vi "sub_rplidar_main.vi"(8 "error in":errorcluster) -> (0 "error out":errorcluster)   [LabVIEW 2019]
uses:
  Ctrl/rplidar_cmd.ctl
panel:
  out "buff chart":u32(graph)
  out "dt":u32
  out "i-2":i32
  out "i-1":i32
  out "XY 그래프":cluster{"X":dbl, "Y":dbl}[](graph)
  out "read buffer":string
  out "n in queue":i32
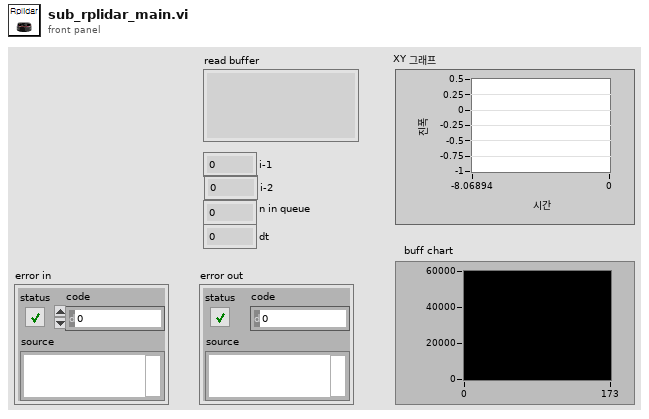
[diagram p1: front panel]
types:
  T1 = typedef "rplidar_cmd.ctl" = enum16{"init", "health", "spin", "scan", "read", "stop", "close"}
  T2 = cluster{"port":refnum<visa-resource-name>, "dt":u32, "update n":u8, "speed":u16, "rate ":u32}
  T3 = typedef "status.ctl" = u16
  T4 = cluster{"AGV":T3, "AGV Estop":T3, "Obstacle":T3, "Heading":T3, "Waypt":T3, "GNSS":T3, "VLP16":T3, "Cam":T3, "RPLidar":T3, "Joystick":T3}
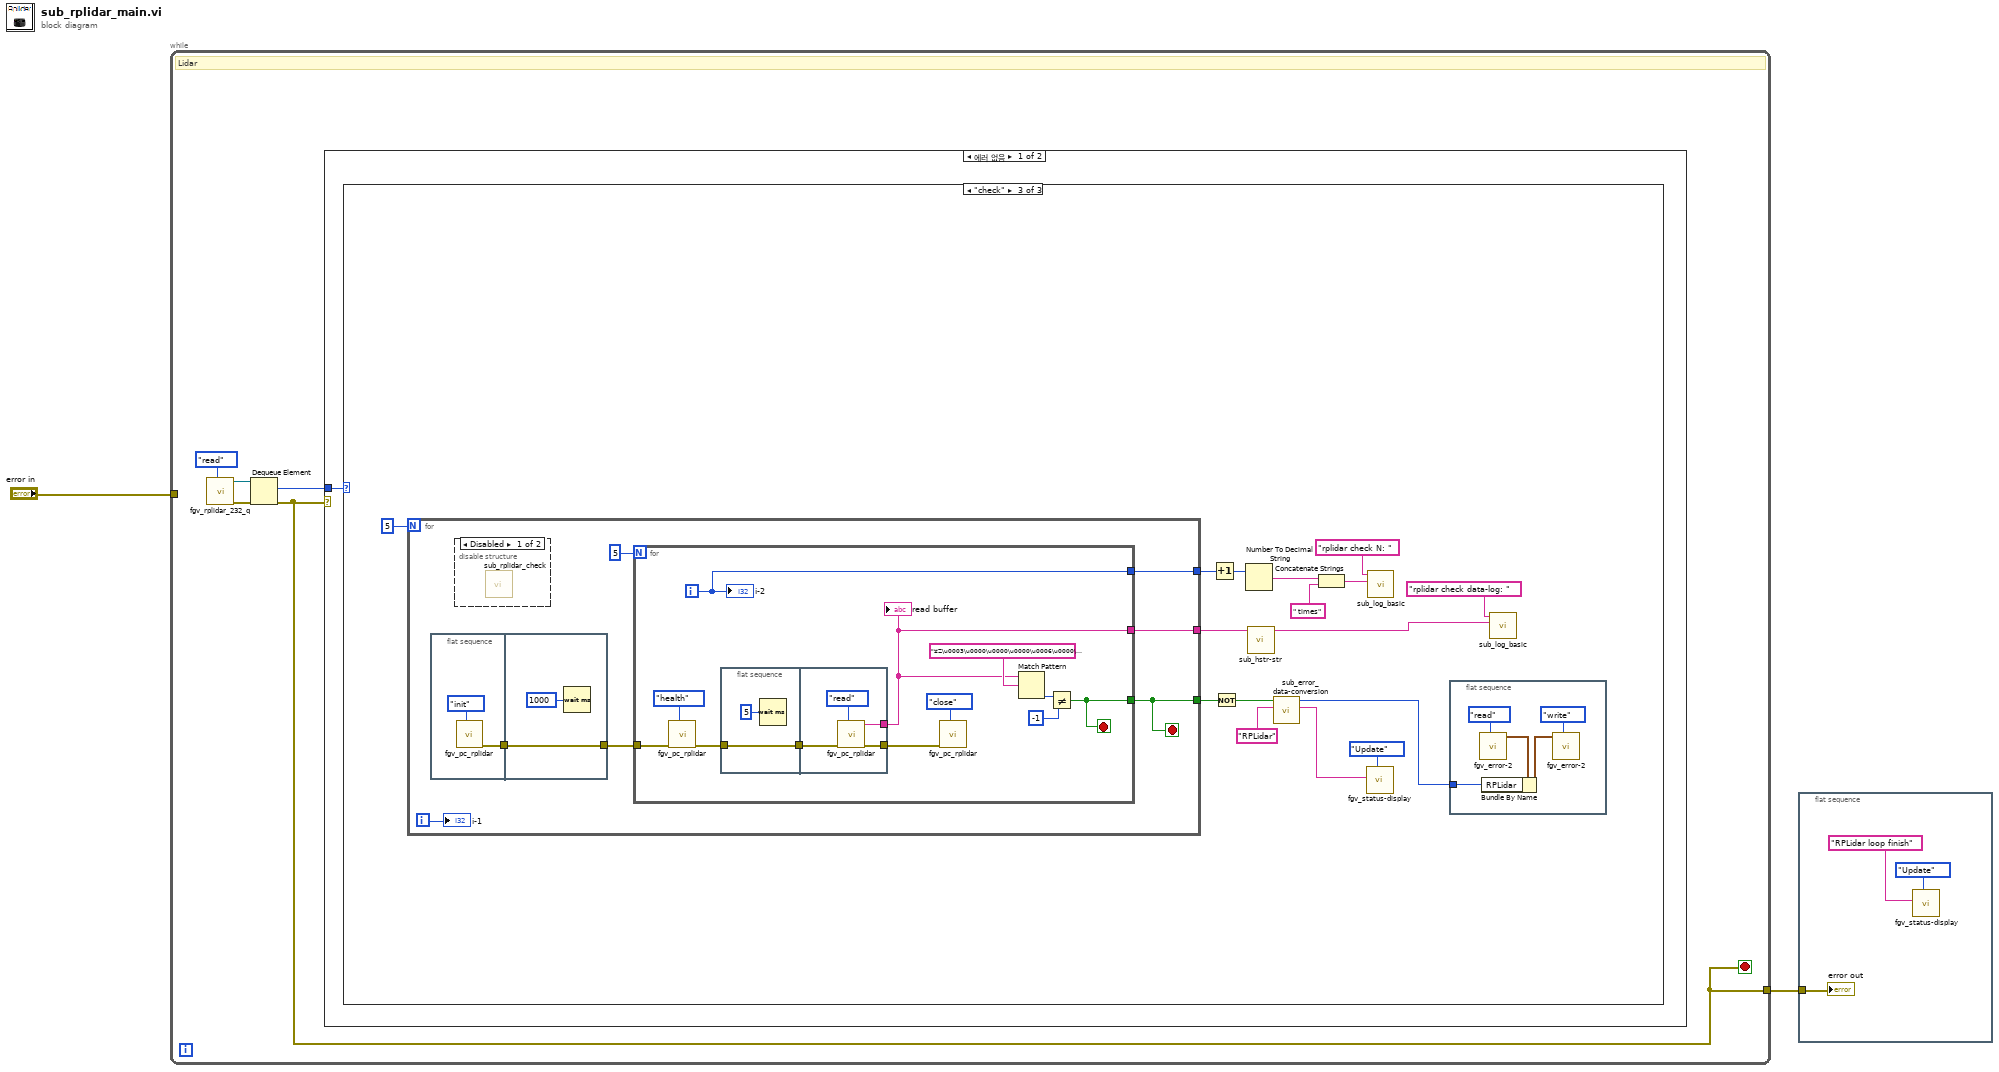
[diagram p0: block diagram]
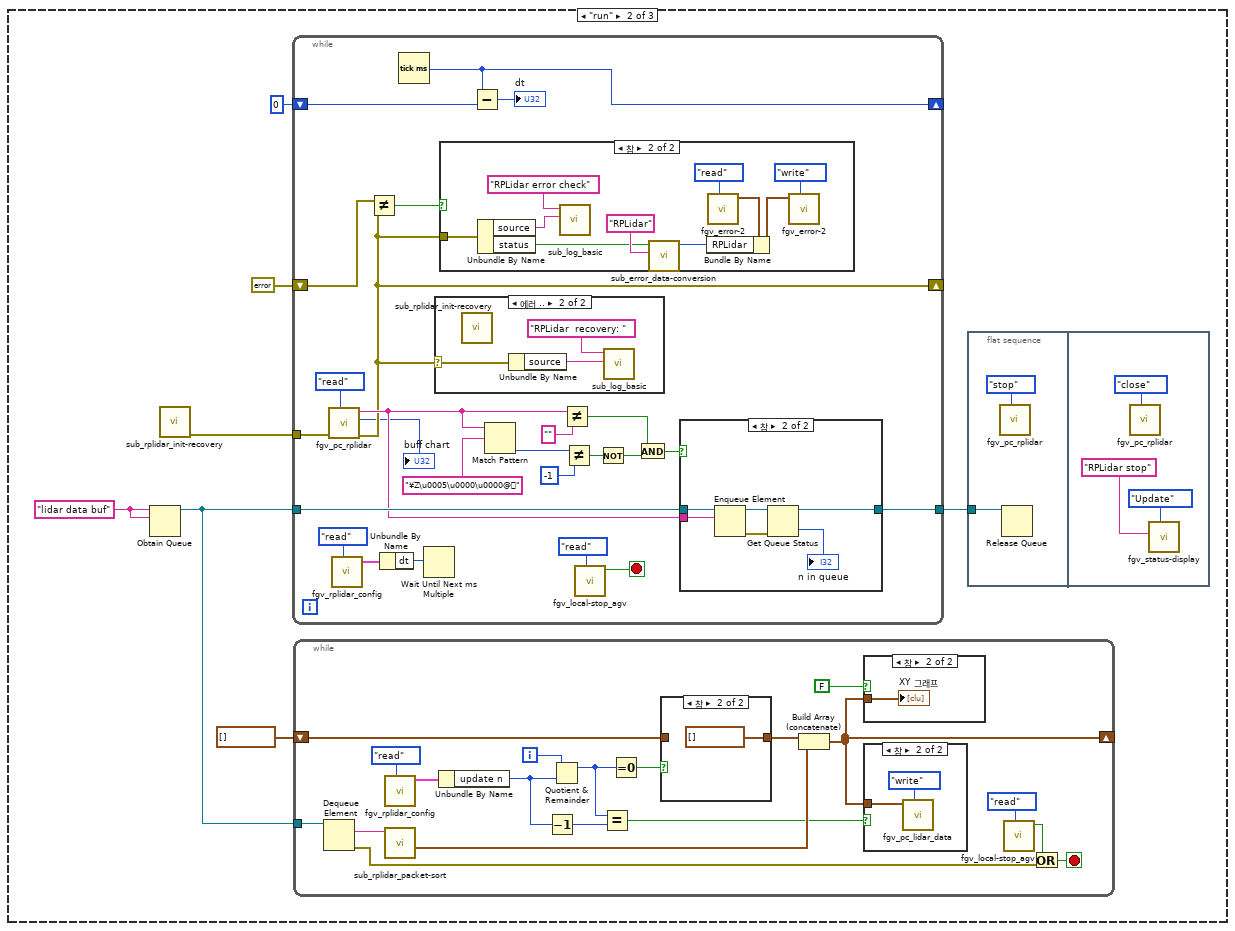
[diagram p3: hidden frame]
diagram:
  n1 = while {
    tunnel: "error in" -> [_]
    tunnel: [w3] -> w1
    stop <- w3 stop-if-true
    # "Lidar"
    n2 = call "fgv_rplidar_232_q.vi"("cmd"=enum16{"create", "write", "read", "close"}."read") -> ("error out"=w7:errorcluster, "queue out"=w4:refnum<queue>)  [unwired: 9 in]
    n3 = Dequeue Element(queue=w4, error in (no error)=w7) -> (element=w6:enum16{"run", "check", "stop"}, error out=w3:errorcluster)  [unwired: 1 in, 2 out]
    n4 = case shown="에러 없음" w3 {
      tunnel: w6 -> [w8 _]
      frame No Error {
        n5 = case shown="\"check\"" w8 {
          frame "stop", Default {
          }
          frame "run" {
            w15 = "lidar data buf" ("name (unnamed)")
            n6 = Obtain Queue(name (unnamed)=w15, element data type=w15) -> (queue out=w11:refnum<queue>)  [unwired: 3 in, 2 out]
            n7 = call "sub_rplidar_init-recovery.vi"() -> ("error out"=w14:errorcluster)  [unwired: 11 in]
            n8 = while {
              tunnel: w14 -> [w68]
              tunnel: w11 -> [w59]
              tunnel: [w58] -> w13
              shift-right: [w49] -> _
              shift-left: errorcluster {"status"=FALSE, "code"=0, "source"=""} ("error out") -> [w51]
              shift-right: [w47] -> _
              shift-left: u32 0 ("millisecond timer value") -> [w48]
              stop <- w55 stop-if-true
              n9 = call "fgv_pc_rplidar.vi"("cmd"=rplidar_cmd."read", "error in"=w68) -> ("error out"=w49:errorcluster, "serial buf"=→"buff chart":u32, "read buffer"=w57:string)  [unwired: 7 in]
              n10 = call "fgv_rplidar_config.vi"("cmd"=enum16{"read", "write"}."read") -> ("RPLidar cfg out"=w53:T2)  [unwired: 9 in, 1 out]
              n11 = Not Equal?(x=w51, y=w49) -> (x != y?=w50:bool)
              n12 = Unbundle By Name(w53) -> ("dt"=w52:u32)
              n13 = Tick Count (ms)() -> (millisecond timer value=w47:u32)
              n14 = Wait Until Next ms Multiple(millisecond multiple=w52) -> ()  [unwired: 1 out]
              n15 = case shown="에러 .." w49 {
                selector: w49 -> [_ w81]
                frame No Error {
                }
                frame Error {
                  n16 = call "sub_rplidar_init-recovery.vi"() -> ()  [unwired: 11 in, 1 out]
                  n17 = Unbundle By Name(w81) -> ("source"=w80:string)
                  n18 = call "sub_log_basic.vi"("desc"=w80, "Title"="RPLidar  recovery: ") -> ()  [unwired: 9 in, 1 out]
                }
              }
              n19 = case shown="참" w50 {
                tunnel: w49 -> [_ w78]
                frame False {
                }
                frame True {
                  n20 = Unbundle By Name(w78) -> ("source"=w70:string, "status"=w71:bool)
                  n21 = call "sub_log_basic.vi"("desc"=w70, "Title"="RPLidar error check") -> ()  [unwired: 9 in, 1 out]
                  n22 = call "sub_error_data-conversion.vi"("name"="RPLidar", "error status"=w71) -> ("error conversion out"=w72:T3)  [unwired: 8 in, 1 out]
                  n23 = call "fgv_error-2.vi"("cmd"=enum16{"init", "read", "write"}."read") -> ("Error cluster out"=w77:T4)  [unwired: 9 in, 1 out]
                  n24 = Bundle By Name(cluster=w77, "RPLidar"=w72) -> (w76:T4)
                  n25 = call "fgv_error-2.vi"("cmd"=enum16{"init", "read", "write"}."write", "Error cluster"=w76) -> ()  [unwired: 8 in, 2 out]
                }
              }
              n26 = Subtract(x=w47, y=w48) -> (x-y=→"dt":u32)
              n27 = Match Pattern(string=w57, regular expression="¥Z\u0005\u0000\u0000@") -> (offset past match=w67:i32)  [unwired: 1 in, 3 out]
              n28 = Not Equal?(x=w57, y="") -> (x != y?=w60:bool)
              n29 = Not Equal?(x=w67, y=-1) -> (x != y?=w64:bool)
              n30 = call "fgv_local-stop_agv.vi"("cmd"=enum16{"ini", "read", "stop"}."read") -> ("stop status"=w55:bool)  [unwired: 10 in]
              n31 = Not(x=w64) -> (.not. x?=w62:bool)
              n32 = And(x=w60, y=w62) -> (x .and. y?=w61:bool)
              n33 = case shown="참" w61 {
                tunnel: w59 -> [w83 w89]
                tunnel: [w83 w86] -> w58
                tunnel: w57 -> [_ w87]
                frame False {
                }
                frame True {
                  n34 = Enqueue Element(queue=w89, element=w87) -> (queue out=w88:refnum<queue>, error out=w85:errorcluster)  [unwired: 2 in, 1 out]
                  n35 = Get Queue Status(queue=w88, error in (no error)=w85) -> (queue out=w86:refnum<queue>, # elements in queue=→"n in queue":i32)  [unwired: 1 in, 6 out]
                }
              }
            }
            n36 = while {
              shift-right: [w25] -> _
              shift-left: cluster{dbl, dbl}[] [] -> [w29]
              tunnel: w11 -> [w34]
              i -> [w28]
              stop <- w32 stop-if-true
              n37 = Dequeue Element(queue=w34) -> (element=w31:string, error out=w33:errorcluster)  [unwired: 2 in, 2 out]
              n38 = call "fgv_rplidar_config.vi"("cmd"=enum16{"read", "write"}."read") -> ("RPLidar cfg out"=w21:T2)  [unwired: 9 in, 1 out]
              n39 = call "sub_rplidar_packet-sort.vi"("rplidar data str"=w31) -> ("xydata"=w26:cluster{"x":dbl, "y":dbl}[])  [unwired: 8 in, 2 out]
              n40 = Unbundle By Name(w21) -> ("update n"=w20:u8)
              n41 = Decrement(x=w20) -> (x-1=w19:u8)
              n42 = Quotient & Remainder(x=w28, y=w20) -> (x-y*floor(x/y)=w18:i32)  [unwired: 1 out]
              n43 = Equal?(x=w18, y=w19) -> (x = y?=w17:bool)
              n44 = Equal To 0?(x=w18) -> (x = 0?=w27:bool)
              n45 = case shown="참" w27 {
                tunnel: [w38 cluster{dbl, dbl}[] []] -> w30
                tunnel: w29 -> [w38 _]
                frame False {
                }
                frame True {
                }
              }
              n46 = Build Array (concatenate)(w30, w26) -> (w25:cluster{"x":dbl, "y":dbl}[])
              n47 = case shown="참" FALSE {
                tunnel: w25 -> [_ w35]
                frame False {
                }
                frame True {
                  "XY 그래프" <- w35
                }
              }
              n48 = case shown="참" w17 {
                tunnel: w25 -> [_ w36]
                frame False {
                }
                frame True {
                  n49 = call "fgv_pc_lidar_data.vi"("cmd"=enum16{"init", "read", "write"}."write", "Lidar array in"=w36) -> ()  [unwired: 9 in, 1 out]
                }
              }
              n50 = call "fgv_local-stop_agv.vi"("cmd"=enum16{"ini", "read", "stop"}."read") -> ("stop status"=w23:bool)  [unwired: 10 in]
              n51 = Or(x=w23, y=w33) -> (x .or. y?=w32:bool)
            }
            n52 = flat-sequence {
              tunnel: w13 -> [w40]
              frame #0 {
                n53 = call "fgv_pc_rplidar.vi"("cmd"=rplidar_cmd."stop") -> ()  [unwired: 8 in, 3 out]
                n54 = Release Queue(queue=w40) -> ()  [unwired: 2 in, 3 out]
              }
              frame #1 {
                n55 = call "fgv_pc_rplidar.vi"("cmd"=rplidar_cmd."close") -> ()  [unwired: 8 in, 3 out]
                n56 = call "fgv_status-display.vi"("Mode"=enum16{"Initial", "Update", "Clear"}."Update", "title"="RPLidar stop" ("String in 1")) -> ()  [unwired: 9 in, 1 out]
              }
            }
          }
          frame "check" {
            n57 = for {
              N: 5 -> [_]
              tunnel: [w114] -> w100
              tunnel: [w112] -> w98
              tunnel: [w111] -> w97
              i -> [w113]
              stop <- w114 stop-if-true
              n58 = flat-sequence {
                tunnel: [w137] -> w117
                tunnel: [w139] -> w116
                tunnel: w117 -> [w139]
                frame #0 {
                  n59 = call "fgv_pc_rplidar.vi"("cmd"=rplidar_cmd."init") -> ("error out"=w137:errorcluster)  [unwired: 8 in, 2 out]
                }
                frame #1 {
                  n60 = Wait (ms)(milliseconds to wait=u32 1000) -> ()  [unwired: 1 out]
                }
              }
              n61 = disable-structure shown="Disabled" {
                frame Disabled {
                  n62 = call "sub_rplidar_check.vi"() -> ()  [unwired: 10 in, 2 out]
                }
                frame Enabled {
                }
              }
              n63 = for {
                N: 5 -> [_]
                tunnel: [w120] -> w114
                tunnel: w116 -> [w124]
                tunnel: [w119] -> w112
                tunnel: [w118] -> w111
                i -> [w118]
                stop <- w120 stop-if-true
                n64 = call "fgv_pc_rplidar.vi"("cmd"=rplidar_cmd."health", "error in"=w124) -> ("error out"=w125:errorcluster)  [unwired: 7 in, 2 out]
                n65 = flat-sequence {
                  tunnel: w125 -> [w131]
                  tunnel: [w131] -> w129
                  tunnel: [w134] -> w121
                  tunnel: [w133] -> w119
                  tunnel: w129 -> [w135]
                  frame #0 {
                    n66 = Wait (ms)(milliseconds to wait=u32 5) -> ()  [unwired: 1 out]
                  }
                  frame #1 {
                    n67 = call "fgv_pc_rplidar.vi"("cmd"=rplidar_cmd."read", "error in"=w135) -> ("error out"=w134:errorcluster, "read buffer"=w133:string)  [unwired: 7 in, 1 out]
                  }
                }
                n68 = call "fgv_pc_rplidar.vi"("cmd"=rplidar_cmd."close", "error in"=w121) -> ()  [unwired: 7 in, 3 out]
                n69 = Match Pattern(string=w119, regular expression="¥Z\u0003\u0000\u0000\u0000\u0006\u0000\u0000\u0000") -> (offset past match=w127:i32)  [unwired: 1 in, 3 out]
                n70 = Not Equal?(x=w127, y=-1) -> (x != y?=w120:bool)
                "read buffer" <- w119
                "i-2" <- w118
              }
              "i-1" <- w113
            }
            n71 = Increment(x=w97) -> (x+1=w96:i32)
            n72 = Not(x=w100) -> (.not. x?=w99:bool)
            n73 = Number To Decimal String(number=w96) -> (decimal integer string=w95:string)  [unwired: 1 in]
            n74 = call "sub_hstr-str.vi"("h-str"=w98) -> ("h2n-str"=w90:string)  [unwired: 10 in]
            n75 = call "sub_error_data-conversion.vi"("name"="RPLidar", "error status"=w99) -> ("check result string"=w104:string, "error conversion out"=w103:T3)  [unwired: 8 in]
            n76 = Concatenate Strings(w95, " times" ("문자열")) -> (w93:string)
            n77 = call "fgv_status-display.vi"("Mode"=enum16{"Initial", "Update", "Clear"}."Update", "title"=w104) -> ()  [unwired: 9 in, 1 out]
            n78 = call "sub_log_basic.vi"("desc"=w93, "Title"="rplidar check N: ") -> ()  [unwired: 9 in, 1 out]
            n79 = flat-sequence {
              tunnel: w103 -> [w108]
              frame #0 {
                n80 = call "fgv_error-2.vi"("cmd"=enum16{"init", "read", "write"}."read") -> ("Error cluster out"=w109:T4)  [unwired: 9 in, 1 out]
                n81 = Bundle By Name(cluster=w109, "RPLidar"=w108) -> (w110:T4)
                n82 = call "fgv_error-2.vi"("cmd"=enum16{"init", "read", "write"}."write", "Error cluster"=w110) -> ()  [unwired: 8 in, 2 out]
              }
            }
            n83 = call "sub_log_basic.vi"("desc"=w90, "Title"="rplidar check data-log: ") -> ()  [unwired: 9 in, 1 out]
          }
        }
      }
      frame Error {
      }
    }
  }
  n84 = flat-sequence {
    tunnel: w1 -> [w142]
    frame #0 {
      n85 = call "fgv_status-display.vi"("Mode"=enum16{"Initial", "Update", "Clear"}."Update", "title"="RPLidar loop finish" ("String in 1")) -> ()  [unwired: 9 in, 1 out]
      "error out" <- w142
    }
  }
